vi "F2_Read_Config.vi"(4 "error in (no error)":errorcluster, 7 "Config Refnum":T1) -> (0 "error out":errorcluster, 2 "All Found?":bool, 3 "refnum out":T1)   [LabVIEW 2015]
uses:
  <vilib>/Utility/config.llb/Config Data RefNum.ctl
  <vilib>/Utility/config.llb/Read Key (I32).vi
  Systems/Secondary Filter/GSP_F2_Global.vi
  <vilib>/Utility/config.llb/Read Key (Double).vi
  <vilib>/Utility/config.llb/NI_LVConfig.lvlib
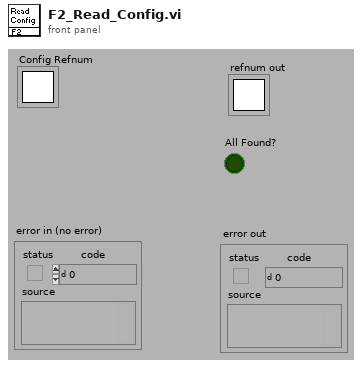
[diagram p1: front panel]
types:
  T1 = typedef "NI_LVConfig.lvlib/Config Data RefNum.ctl" = refnum<k1>
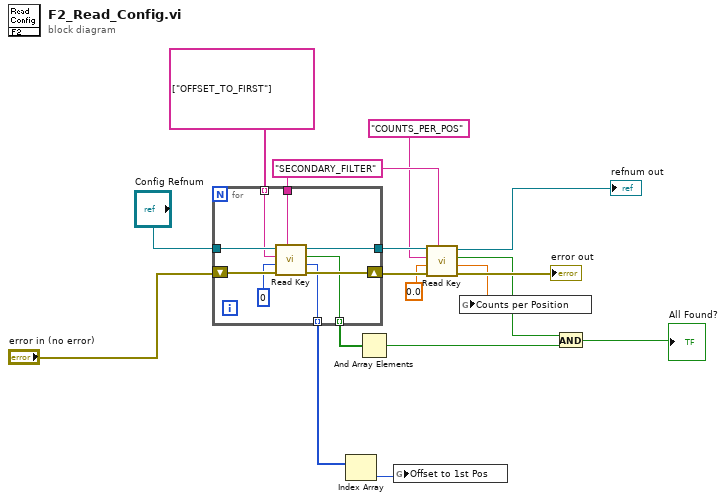
[diagram p0: block diagram]
diagram:
  w12 = "SECONDARY_FILTER"
  n1 = for {
    tunnel: "Config Refnum" -> [w25]
    shift-right: [w24] -> w13
    shift-left: "error in (no error)" -> [w26]
    tunnel: [w23] -> w14
    tunnel: string[] ["OFFSET_TO_FIRST"] -> [w22] mode=indexing
    tunnel: w12 -> [w21]
    tunnel: [w19] -> w8 mode=indexing
    tunnel: [w18] -> w7 mode=indexing
    n2 = call-poly <vilib>:"Read Key.vi"("section"=w21, "error in (no error)"=w26, "default value"=0, "key"=w22, "refnum"=w25) -> ("error out"=w24:errorcluster, "value"=w19:i32, "found?"=w18:bool, "refnum out"=w23:T1)  [unwired: 3 in]
  }
  n3 = Index Array(array=w8) -> (element=w1:i32)  [unwired: 1 in]
  n4 = And Array Elements(Boolean array=w7) -> (logical AND=w5:bool)
  n5 = global write "GSP_F2_Global.vi" "Offset to 1st Pos"(w1) -> ()
  n6 = call-poly <vilib>:"Read Key.vi"("section"=w12, "error in (no error)"=w13, "default value"=0.0, "key"="COUNTS_PER_POS", "refnum"=w14) -> ("error out"=→"error out":errorcluster, "value"=w3:dbl, "found?"=w6:bool, "refnum out"=→"refnum out":T1)  [unwired: 3 in]
  n7 = global write "GSP_F2_Global.vi" "Counts per Position"(w3) -> ()
  n8 = And(x=w6, y=w5) -> (x .and. y?=→"All Found?":bool)
